vi "Saturated Add.vi"(10 "Sizes":i16[](array[numeric])) -> (2 "Sum":i16)   [LabVIEW 2013, in "Divider.lvclass"]
doc: "Copyright 2018, Wiebe Walstra, wiebe@carya.nl."
uses:
  Divider.lvclass
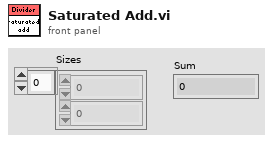
[diagram p1: front panel]
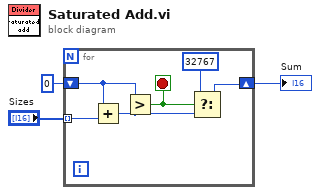
[diagram p0: block diagram]
diagram:
  n1 = for {
    tunnel: "Sizes" -> [w9] mode=indexing
    shift-right: [w5] -> w1
    shift-left: i16 0 -> [w8]
    stop <- w4 stop-if-true
    n2 = Add(x=w8, y=w9) -> (x+y=w7:i16)
    n3 = Greater?(x=w8, y=w7) -> (0:w4:bool)
    n4 = Select(t=i16 32767 ("f"), s=w4, f=w7) -> (s? t:f=w5:i16)
  }
  "Sum" <- w1
